vi "Get File Size.vi"(8 "error in (no error)":errorcluster, 11 "Log File in":refnum<class "Log File.lvclass">) -> (0 "error out":errorcluster, 2 "size (in bytes)":i64, 3 "Log File out":refnum<class "Log File.lvclass">)   [LabVIEW 2015, in "Log File.lvclass"]
uses:
  Log File.lvclass
  Log File.lvclass/Log File.ctl
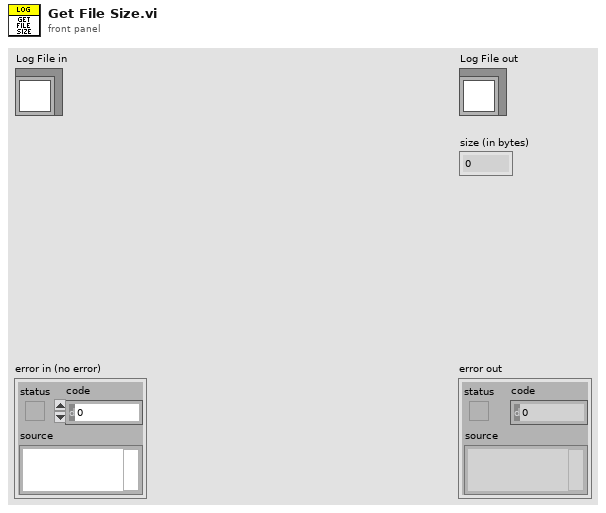
[diagram p1: front panel]
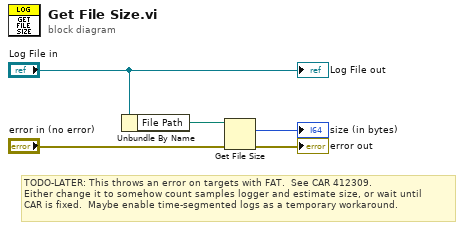
[diagram p0: block diagram]
diagram:
  # "TODO-LATER: This throws an error on targets with FAT.  See CAR 412309.\nEither change it to somehow count samples logger and estimate size, or wait until\nCAR is fixed.  Maybe enable time-segmented logs as a temporary workaround."
  n1 = Unbundle By Name("Log File in") -> ("File Path"=w2:path)
  n2 = Get File Size(file=w2, error in="error in (no error)") -> (size (in bytes)=→"size (in bytes)":i64, 0:→"error out":errorcluster)  [unwired: 1 out]
  "Log File out" <- "Log File in"
